vi "Check Files.vi"(8 "error in (no error)":errorcluster, 11 "Sequence Directory In":path) -> (0 "error out":errorcluster, 2 "Files Valid?":bool, 3 "Sequence Directory Out":path)   [LabVIEW 2015]
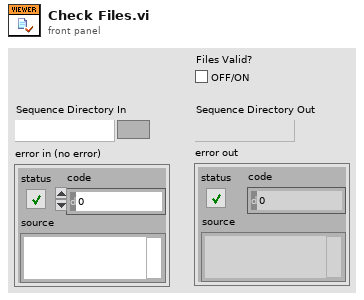
[diagram p1: front panel]
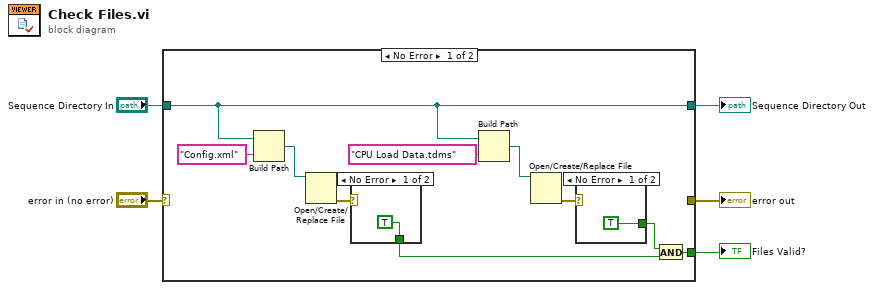
[diagram p0: block diagram]
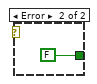
[diagram p2: hidden frame]
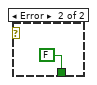
[diagram p3: hidden frame]
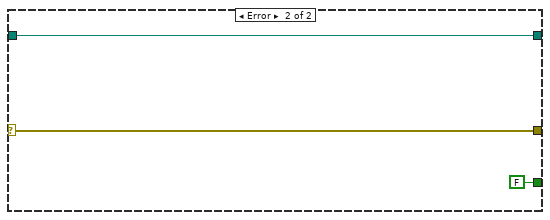
[diagram p4: hidden frame]
diagram:
  n1 = case shown="No Error" "error in (no error)" {
    selector: "error in (no error)" -> [_ w22]
    tunnel: "Sequence Directory In" -> [w11 w21]
    tunnel: [w11 w21] -> w3
    tunnel: [_ w22] -> w2
    tunnel: [w6 FALSE] -> w1
    frame No Error {
      n2 = Build Path(base path=w11, name or relative path="Config.xml") -> (appended path=w14:path)
      n3 = Open/Create/Replace File(file path (use dialog)=w14) -> (error out=w10:errorcluster)  [unwired: 5 in, 2 out]
      n4 = case shown="No Error" w10 {
        tunnel: [TRUE FALSE] -> w7
        frame No Error {
        }
        frame Error {
        }
      }
      n5 = Build Path(base path=w11, name or relative path="CPU Load Data.tdms") -> (appended path=w12:path)
      n6 = Open/Create/Replace File(file path (use dialog)=w12) -> (error out=w9:errorcluster)  [unwired: 5 in, 2 out]
      n7 = case shown="No Error" w9 {
        tunnel: [TRUE FALSE] -> w8
        frame No Error {
        }
        frame Error {
        }
      }
      n8 = And(x=w8, y=w7) -> (x .and. y?=w6:bool)
    }
    frame Error {
    }
  }
  "error out" <- w2
  "Sequence Directory Out" <- w3
  "Files Valid?" <- w1
